vi "CI Project Builder.vi"() -> ()   [LabVIEW 2014, in "CI Project Builder.lvlib"]
doc: "This is the main VI for the configuration editor."
uses:
  CI Project Builder.lvlib
  Controls/StateCluster.ctl
  <vilib>/ni/Configuration Framework/Node/NodeRef.ctl
  <vilib>/ni/Configuration Framework/Node/NISE_CEF_Node.lvclass
  <vilib>/ni/Configuration Framework/Node/StandardEvents.ctl
  <vilib>/ni/Configuration Framework/Node/UserEventRef.ctl
  <vilib>/ni/Configuration Framework/Controls/EventCluster.ctl
  <vilib>/ni/Configuration Framework/Node/NodeChangeEvent.ctl
  <vilib>/ni/Configuration Framework/Node/CacheState.ctl
  <vilib>/ni/Configuration Framework/Node/RefreshUIEvent.ctl
  <vilib>/ni/Configuration Framework/Node/StopEvent.ctl
  <vilib>/ni/Configuration Framework/glyph manager/glyph manager.ctl
  <vilib>/picture/picture.llb/imagedata.ctl
  Controls/AddMessage.ctl
  Controls/MoveMessage.ctl
  <vilib>/Utility/error.llb/DialogType.ctl
  <vilib>/ni/AMC/Message Queue.ctl
  <vilib>/ni/AMC/Message.ctl
  <vilib>/ni/Tools/Keyed Array/KeyedArray.ctl
  Classes/CI Project/CI Project.lvclass
  <vilib>/ni/Configuration Framework/class discovery singleton/class discovery singleton methods.ctl
  <vilib>/ni/AMC/Read Termination Message.vi
  <vilib>/ni/AMC/Create Single Message.vi
  <vilib>/ni/AMC/Update Message Routing Info.vi
  <vilib>/ni/AMC/Send Message.vi
  <vilib>/ni/AMC/Globals.vi
  Classes/INI Deserializer/INI Deserializer.lvclass
  <vilib>/ni/AMC/AMC.lvlib
  <vilib>/ni/Configuration Framework/NISE_CEF_TreeControl.lvlib
  <vilib>/ni/Configuration Framework/glyph manager/glyph manager.lvlib
  <vilib>/ni/Configuration Framework/class discovery singleton/class discovery singleton.lvlib
  <vilib>/ni/Tools/Keyed Array/Tools_KeyedArray.lvlib
panel:
  in  "View":string(tree)
  in  "Exit":bool
  # "Continuous Integration Project Builder"
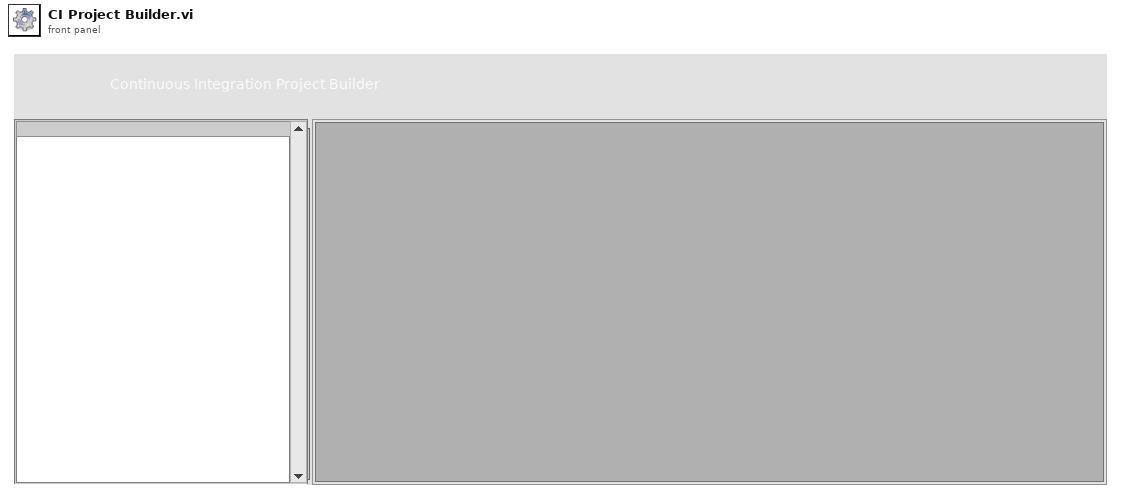
[diagram p1: front panel]
types:
  T1 = typedef "CI Project Builder.lvlib/StateCluster.ctl" = cluster{"root":T2, "unsaved changes":bool, "current path":path, "standard events":T3, "classes path":path, "glyph manager":T9, "Exports Path":path}
  T2 = typedef "NISE_CEF_Node.lvclass/NodeRef.ctl" = refnum<data-value>
  T3 = typedef "NISE_CEF_Node.lvclass/StandardEvents.ctl" = cluster{"user event":T4, "node change":T5, "cache state":T6, "refresh UI":T7, "stop event":T8}
  T4 = typedef "NISE_CEF_Node.lvclass/UserEventRef.ctl" = refnum<user-event>
  T5 = typedef "NISE_CEF_Node.lvclass/NodeChangeEvent.ctl" = refnum<user-event>
  T6 = typedef "NISE_CEF_Node.lvclass/CacheState.ctl" = refnum<user-event>
  T7 = typedef "NISE_CEF_Node.lvclass/RefreshUIEvent.ctl" = refnum<user-event>
  T8 = typedef "NISE_CEF_Node.lvclass/StopEvent.ctl" = refnum<user-event>
  T9 = typedef "glyph manager.lvlib/glyph manager.ctl" = cluster{"search paths":path[], "glyph map":variant, "base glyphs":T10[], "desired overlays":string[]}
  T10 = typedef "imagedata.ctl" = cluster{"image type":i32, "image depth":i32, "image":u8[], "mask":u8[], "colors":u32[], "Rectangle":cluster{"left":i16, "top":i16, "right":i16, "bottom":i16}}
  T11 = typedef "AMC.lvlib/Message Queue.ctl" = refnum<queue>
  T12 = enum32{"Invalid", "Standard", "Closed", "Hidden", "Minimized", "Maximized"}
  T13 = typedef "class discovery singleton.lvlib/class discovery singleton methods.ctl" = enum16{"add search paths", "load class by name", "list available classes", "get class path", "delete cache"}
  T14 = typedef "CI Project Builder.lvlib/AddMessage.ctl" = cluster{"node type":string, "to add to":string}
  T15 = typedef "CI Project Builder.lvlib/MoveMessage.ctl" = cluster{"node ref":T2, "new parent":T2, "Position":i32}
  T16 = typedef "CI Project Builder.lvlib/FilePaths.ctl" = cluster{"glyphs":path, "classes":path}
  T17 = typedef "DialogType.ctl" = u16
  T18 = typedef "NISE_CEF_Node.lvclass/Summary.ctl" = cluster{"ID":string, "parent ID":string, "node type":string, "text":string, "additional text":string, "glyph":string, "depth":i32, "glyph overlay":string}
  T19 = typedef "LVPoint32TypeDef.ctl" = cluster{"Horizontal":i32, "Vertical":i32}
  T20 = cluster{"data name":string, "drag data":variant}[]
  T21 = typedef "NISE_CEF_Node.lvclass/NodeMenuOptions.ctl" = cluster{"removable":bool, "movable":bool, "duplicate":bool}
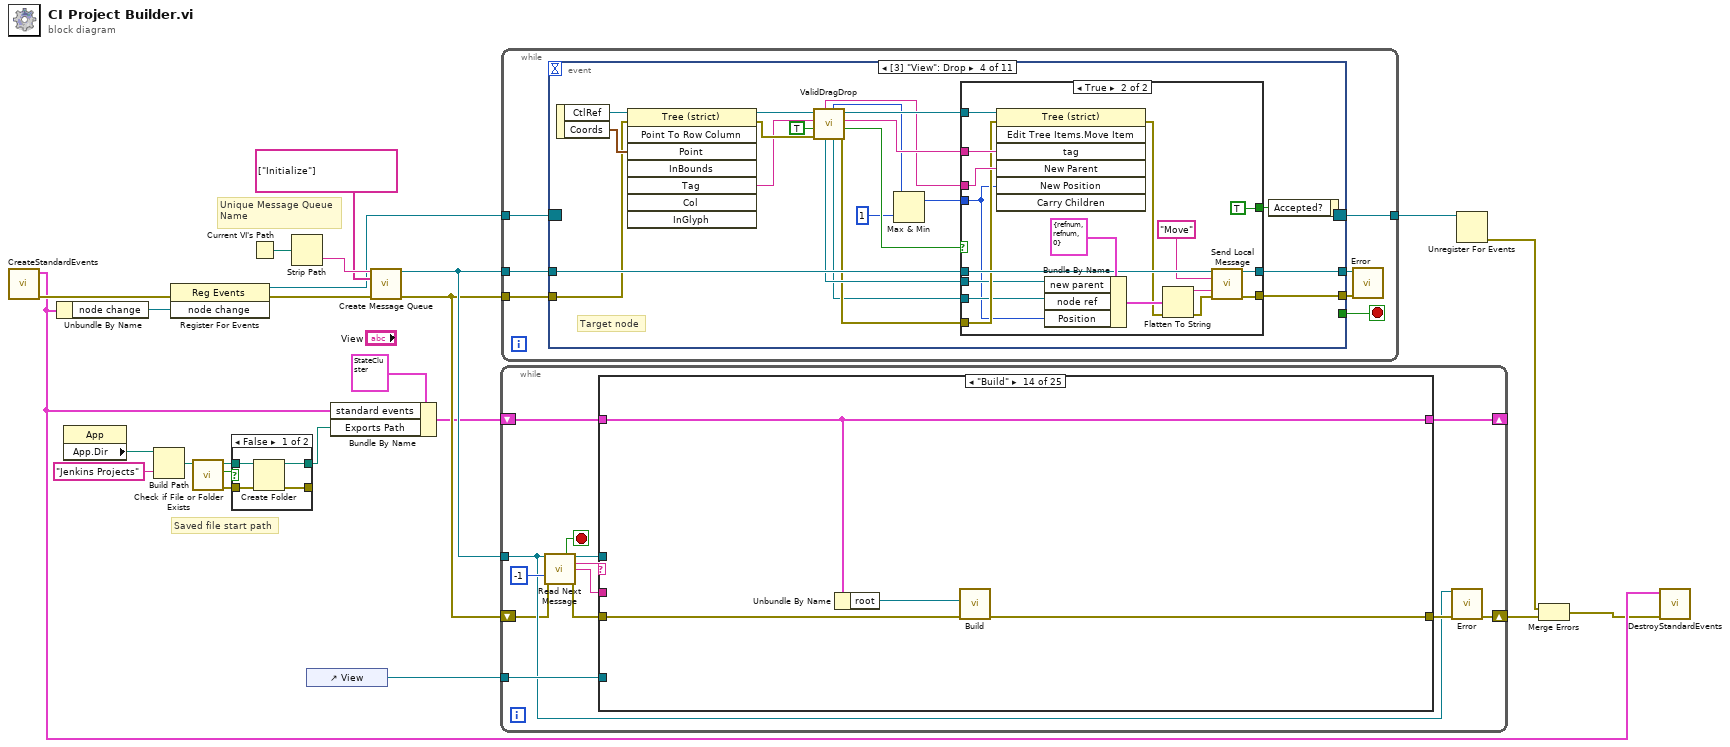
[diagram p0: block diagram]
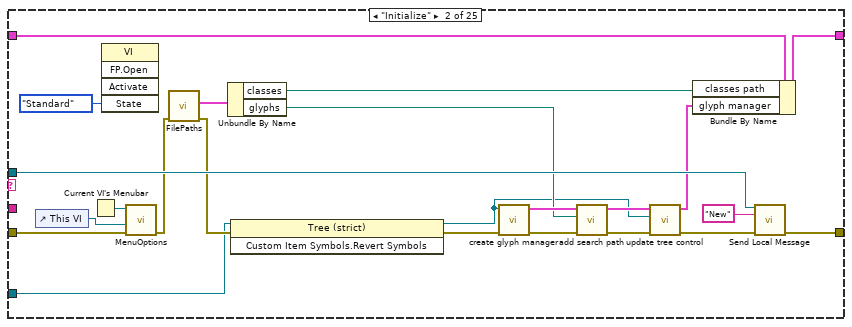
[diagram p4: hidden frame]
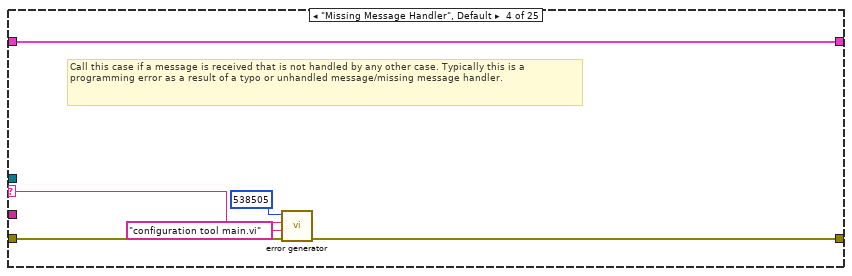
[diagram p6: hidden frame]
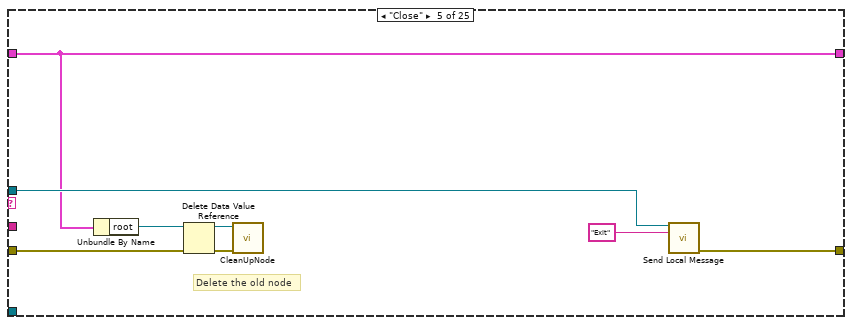
[diagram p7: hidden frame]
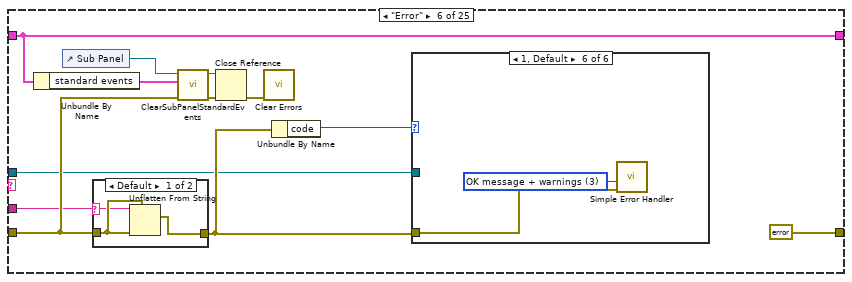
[diagram p8: hidden frame]
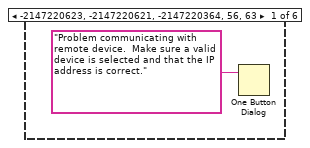
[diagram p10: hidden frame]
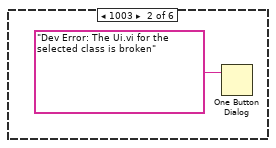
[diagram p11: hidden frame]
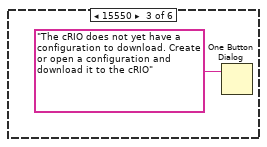
[diagram p12: hidden frame]
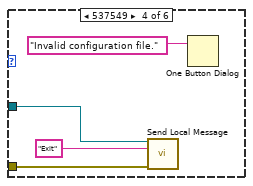
[diagram p13: hidden frame]
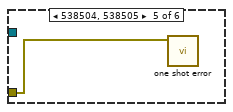
[diagram p14: hidden frame]
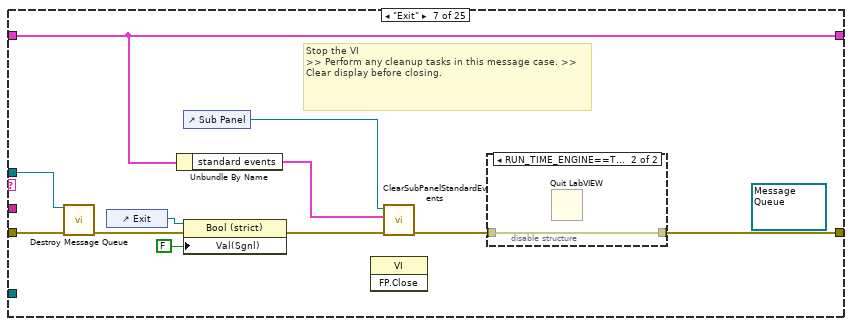
[diagram p15: hidden frame]
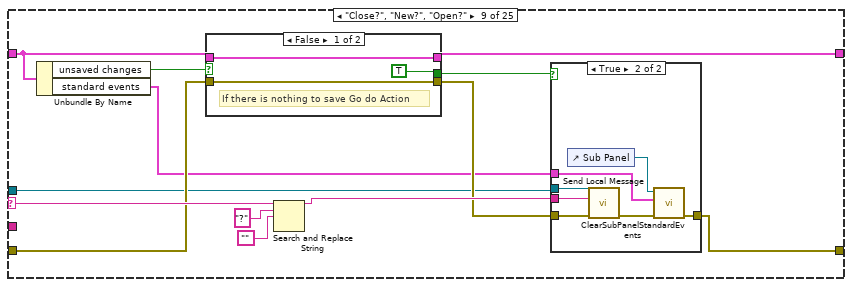
[diagram p18: hidden frame]
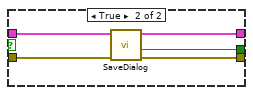
[diagram p19: hidden frame]
diagram:
  # "Saved file start path"
  # "Unique Message Queue Name"
  n1 = call <vilib>:"CreateStandardEvents.vi"() -> ("error out"=w19:errorcluster, "standard events"=w13:T3)  [unwired: 10 in]
  n2 = Unbundle By Name(w13) -> ("node change"=w18:T5)
  n3 = property class="App"() -> ("App.Dir"=w2:path)  [unwired: 2 in, 2 out]
  n4 = Build Path(base path=w2, name or relative path="Jenkins Projects") -> (appended path=w3:path)
  n5 = register-events(error in=w19, w18) -> (reference out=w12:refnum<event-registration>, error out=w17:errorcluster)  [unwired: 1 in]
  n6 = call <vilib>:"Check if File or Folder Exists.vi"("path"=w3) -> ("error out"=w4:errorcluster, "file or folder exists?"=w6:bool, "dup path"=w5:path)  [unwired: 8 in]
  n7 = case shown="False" w6 {
    tunnel: w5 -> [w28 w30]
    tunnel: [w27 w30] -> w1
    tunnel: w4 -> [w26 w29]
    tunnel: [w25 w29] -> _
    frame False {
      n8 = Create Folder(path (use dialog)=w28, error in=w26) -> (created path=w27:path, error out=w25:errorcluster)  [unwired: 1 in, 1 out]
    }
    frame True {
    }
  }
  n9 = Current VI's Path() -> (path=w23:path)
  n10 = Strip Path(path=w23) -> (name=w24:string)  [unwired: 1 out]
  n11 = control-ref of="View"() -> (w11:refnum<vi>)
  n12 = Bundle By Name(cluster=T1 {"root"=refnum, "unsaved changes"=FALSE, "current path"=path "", "standard events"={"user event"=refnum, "node change"=refnum, "cache state"=refnum, "refresh UI"=refnum, "stop event"=refnum}, "classes path"=path "", "glyph manager"={"search paths"=[], "glyph map"=variant, "base glyphs"=[], "desired overlays"=[]}, "Exports Path"=path ""}, "standard events"=w13, "Exports Path"=w1) -> (w15:T1)
  n13 = call <vilib>:"Create Message Queue.vi"("message queue name"=w24, "initial message names"=string[] ["Initialize"], "error in"=w17) -> ("message queue out"=w21:T11, "error out"=w20:errorcluster)  [unwired: 11 in]
  n14 = while "Message Processor" {
    shift-right: [w34] -> w14
    shift-left: w20 -> [w32]
    tunnel: w21 -> [w33]
    shift-right: [w40] -> _
    shift-left: w15 -> [w39]
    tunnel: w11 -> [w37]
    stop <- w43 stop-if-true
    n15 = call <vilib>:"Read Next Message.vi"("message queue in"=w33, "timeout (1 ms)"=-1, "error in"=w32) -> ("exit process?"=w43:bool, "message queue out"=w38:T11, "message name"=w42:string, "message value"=w41:string, "error out"=w31:errorcluster)  [unwired: 5 in, 3 out]
    n16 = case shown="\"Build\"" w42 {
      selector: w42 -> [_ _ _ w72 _ _ _ _ w135 _ _ _ _ _ _ _ _ w284 _ _ _ _ _ _ _]
      tunnel: w41 -> [_ _ _ _ _ w87 _ _ _ _ _ _ _ _ _ w251 w262 w282 w335 w361 _ _ w401 w424 w429]
      tunnel: w31 -> [w45 w68 w70 w75 w79 w90 w121 w125 w128 w157 w175 w204 w219 w224 w227 w232 w261 w287 w337 w360 w382 w391 w400 w422 w430]
      tunnel: [w45 w64 w70 w73 w83 errorcluster {"status"=FALSE, "code"=0, "source"=""} ("error out") w113 w125 w138 w169 w171 w206 w221 w223 w227 w245 w265 w290 w339 w357 w376 w387 w397 w417 w428] -> w35
      tunnel: [w44 w60 w69 w76 w81 w94 w112 w124 w130 w167 w176 w209 w220 w225 w226 w242 w258 w291 w338 w354 w373 w390 w396 w413 w431] -> w40
      tunnel: w39 -> [w44 w61 w69 w76 w81 w94 w112 w124 w131 w164 w177 w201 w218 w225 w226 w233 w259 w291 w331 w362 w385 w390 w396 w425 w431]
      tunnel: w38 -> [_ w63 _ _ w82 w85 w120 _ w126 w168 w173 w205 _ _ _ _ _ w285 _ _ _ _ w393 w416 w427]
      tunnel: w37 -> [_ w47 _ _ _ _ _ _ _ _ _ _ _ _ _ w243 w254 w279 w333 w355 w374 _ _ _ _]
      frame "------------Generic Operations------------" {
        # "Dummy case to add a seperation in the Case Structure menu"
      }
      frame "Initialize" {
        n17 = control-ref of="This VI"() -> (w67:refnum<vi>)
        n18 = Current VI's Menubar() -> (w66:refnum<k9>)
        n19 = invoke class="VI" method="FP.Open"("State"=T12."Standard") -> ()  [unwired: 4 in, 5 out]
        n20 = call "MenuOptions.vi"("error in"=w68, "VI ref"=w67, "menu ref in"=w66) -> ("error out"=w59:errorcluster)  [unwired: 7 in, 1 out]
        n21 = call "FilePaths.vi"("error in"=w59) -> ("error out"=w50:errorcluster, "paths"=w62:T16)  [unwired: 9 in]
        n22 = Unbundle By Name(w62) -> ("classes"=w58:path, "glyphs"=w52:path)
        n23 = invoke class="Tree (strict)" method="Custom Item Symbols.Revert Symbols"(reference=w47, error in=w50) -> (reference out=w48:refnum<vi>, error out=w49:errorcluster)  [unwired: 1 in, 1 out]
        n24 = call <vilib>:"create glyph manager.vi"("error in"=w49, "tree ref (for default symbols)"=w48) -> ("error out"=w57:errorcluster, "glyph manager"=w56:T9)  [unwired: 8 in]
        n25 = call <vilib>:"add search path.vi"("error in"=w57, "search path"=w52, "glyph manager in"=w56) -> ("error out"=w55:errorcluster, "glyph manager out"=w54:T9)  [unwired: 7 in]
        n26 = call <vilib>:"update tree control.vi"("error in"=w55, "tree reference"=w48, "glyph manager in"=w54) -> ("error out"=w53:errorcluster, "glyph manager out"=w51:T9)  [unwired: 7 in]
        n27 = Bundle By Name(cluster=w61, "classes path"=w58, "glyph manager"=w51) -> (w60:T1)
        n28 = call <vilib>:"Send Local Message.vi"("message queue in"=w63, "message name"="New" ("Message Name"), "error in"=w53) -> ("error out"=w64:errorcluster)  [unwired: 10 in, 2 out]
      }
      frame "", "Idle" {
      }
      frame "Missing Message Handler", Default {
        # "Call this case if a message is received that is not handled by any other case. Typically this is a programming error as a result of a typo or unhandled message/missing message handler."
        n29 = call <vilib>:"error generator.vi"("error in"=w75, "source"="configuration tool main.vi", "append error message"=w72, "error code (0)"=538505) -> ("error out"=w73:errorcluster)  [unwired: 5 in]
      }
      frame "Close" {
        # "Delete the old node"
        n30 = Unbundle By Name(w81) -> ("root"=w80:T2)
        n31 = Delete Data Value Reference(data value reference=w80, error in=w79) -> (data value=w78:refnum<class "NISE_CEF_Node.lvclass">, error out=w77:errorcluster)
        n32 = call-dynamic "CleanUpNode.vi"("error in (no error)"=w77, "NISE_CEF_Node in"=w78) -> ()  [unwired: 8 in, 2 out]
        n33 = call <vilib>:"Send Local Message.vi"("message queue in"=w82, "message name"="Exit") -> ("error out"=w83:errorcluster)  [unwired: 11 in, 2 out]
      }
      frame "Error" {
        n34 = Unbundle By Name(w94) -> ("standard events"=w86:T3)
        n35 = control-ref of="Sub Panel"() -> (w93:refnum<vi>)
        n36 = case shown="Default" w87 {
          selector: w87 -> [w98 _]
          tunnel: w90 -> [w99 w100]
          tunnel: [w97 w100] -> w89
          frame Default {
            n37 = Unflatten From String(type=w99, binary string=w98, error in (no error)=w99) -> (value=w97:errorcluster)  [unwired: 2 in, 2 out]
          }
          frame "" {
          }
        }
        n38 = call <vilib>:"ClearSubPanelStandardEvents.vi"("error in"=w90, "standard events"=w86, "sub panel ref in"=w93) -> ("error out"=w92:errorcluster, "sub panel ref out"=w91:refnum<vi>)  [unwired: 7 in]
        n39 = Close Reference(reference=w91, error in (no error)=w92) -> (error out=w88:errorcluster)
        n40 = call <vilib>:"Clear Errors.vi"("error in (no error)"=w88) -> ()  [unwired: 5 in, 2 out]
        n41 = Unbundle By Name(w89) -> ("code"=w95:i32)
        n42 = case shown="1, Default" w95 {
          tunnel: w85 -> [_ _ _ w106 _ _]
          tunnel: w89 -> [_ _ _ w105 w108 w110]
          frame -2147220623, -2147220621, -2147220364, 56, 63 {
            n43 = One Button Dialog(message="Problem communicating with remote device.  Make sure a valid device is selected and that the IP address is correct.") -> ()  [unwired: 1 in, 1 out]
          }
          frame 1003 {
            n44 = One Button Dialog(message="Dev Error: The Ui.vi for the selected class is broken") -> ()  [unwired: 1 in, 1 out]
          }
          frame 15550 {
            n45 = One Button Dialog(message="The cRIO does not yet have a configuration to download. Create or open a configuration and download it to the cRIO") -> ()  [unwired: 1 in, 1 out]
          }
          frame 537549 {
            n46 = call <vilib>:"Send Local Message.vi"("message queue in"=w106, "message name"="Exit", "error in"=w105) -> ()  [unwired: 10 in, 3 out]
            n47 = One Button Dialog(message="Invalid configuration file.") -> ()  [unwired: 1 in, 1 out]
          }
          frame 538504, 538505 {
            n48 = call <vilib>:"one shot error.vi"("error in"=w108) -> ()  [unwired: 11 in]
          }
          frame 1, Default {
            w109 = T17 3 items=["no dialog", "OK message", "continue or stop message", "OK message + warnings", "continue/stop + warnings"] ("type of dialog (OK msg:1)")
            n49 = call <vilib>:"Simple Error Handler.vi"("type of dialog (OK msg:1)"=w109, "error in (no error)"=w110) -> ()  [unwired: 8 out]
          }
        }
      }
      frame "Exit" {
        (unwired) T11 refnum ("message queue out")
        # "Stop the VI                                                                             >> Perform any cleanup tasks in this message case. >> Clear display before closing."
        n50 = call <vilib>:"Destroy Message Queue.vi"("message queue in"=w120, "error in"=w121) -> ("error out"=w117:errorcluster)  [unwired: 11 in, 2 out]
        n51 = control-ref of="Exit"() -> (w119:refnum<vi>)
        n52 = Unbundle By Name(w112) -> ("standard events"=w111:T3)
        n53 = control-ref of="Sub Panel"() -> (w116:refnum<vi>)
        n54 = property class="Bool (strict)"(reference=w119, error in=w117, "Val(Sgnl)"=FALSE ("Exit")) -> (error out=w115:errorcluster)  [unwired: 1 out]
        n55 = invoke class="VI" method="FP.Close"() -> ()  [unwired: 3 in, 3 out]
        n56 = call <vilib>:"ClearSubPanelStandardEvents.vi"("error in"=w115, "standard events"=w111, "sub panel ref in"=w116) -> ("error out"=w114:errorcluster)  [unwired: 7 in, 1 out]
        n57 = disable-structure shown="RUN_TIME_ENGINE==True" {
          disable-tunnel: [w122 w123] -> w113
          disable-tunnel: w114 -> [w122 w123]
          frame condition #0 (active) {
          }
          frame condition #1 {
            n58 = Quit LabVIEW() -> ()  [unwired: 1 in]
          }
        }
      }
      frame "------------Menu Operations--------------" {
        # "Dummy case to add a seperation in the Case Structure menu"
      }
      frame "Close?", "New?", "Open?" {
        n59 = Unbundle By Name(w131) -> ("unsaved changes"=w133:bool, "standard events"=w127:T3)
        n60 = case shown="False" w133 {
          tunnel: [TRUE ("SaveFlag") w146] -> w132
          tunnel: w131 -> [w140 w145]
          tunnel: [w140 w144] -> w130
          tunnel: w128 -> [w139 w143]
          tunnel: [w139 w142] -> w129
          frame False {
            # "If there is nothing to save Go do Action"
          }
          frame True {
            n61 = call "SaveDialog.vi"("error in"=w143, "state in"=w145) -> ("error out"=w142:errorcluster, "new"=w146:bool, "state out"=w144:T1)  [unwired: 7 in]
          }
        }
        n62 = Search and Replace String(input string=w135, search string="?", replace string="") -> (result string=w134:string)  [unwired: 5 in, 3 out]
        n63 = case shown="True" w132 {
          tunnel: w129 -> [w147 w154]
          tunnel: [w147 w150] -> w138
          tunnel: w126 -> [_ w153]
          tunnel: w134 -> [_ w152]
          tunnel: w127 -> [_ w148]
          frame False {
          }
          frame True {
            n64 = control-ref of="Sub Panel"() -> (w149:refnum<vi>)
            n65 = call <vilib>:"Send Local Message.vi"("message queue in"=w153, "message name"=w152, "error in"=w154) -> ("error out"=w151:errorcluster)  [unwired: 10 in, 2 out]
            n66 = call <vilib>:"ClearSubPanelStandardEvents.vi"("error in"=w151, "standard events"=w148, "sub panel ref in"=w149) -> ("error out"=w150:errorcluster)  [unwired: 7 in, 1 out]
          }
        }
      }
      frame "New" {
        # "Delete the old node, if any"
        n67 = Unbundle By Name(w164) -> ("root"=w156:T2, "classes path"=w159:path)
        n68 = Delete Data Value Reference(data value reference=w156) -> (data value=w155:refnum<class "NISE_CEF_Node.lvclass">)  [unwired: 1 in, 1 out]
        n69 = call-dynamic "CleanUpNode.vi"("NISE_CEF_Node in"=w155) -> ()  [unwired: 9 in, 2 out]
        n70 = Build Array(w159) -> (w160:path[])
        n71 = call <vilib>:"class discovery singleton.vi"("error in"=w157, "Plugin Search Paths"=w160, "method"=class_discovery_singleton_methods."add search paths") -> ("error out"=w158:errorcluster)  [unwired: 5 in, 3 out]
        n72 = call-dynamic "Initialize.vi"("error in"=w158, "node in"=refnum<class "CI Project.lvclass"> refnum ("CI Project.lvclass")) -> ("error out"=w163:errorcluster, "data value reference"=w165:T2)  [unwired: 7 in, 1 out]
        n73 = Bundle By Name(cluster=w164, "unsaved changes"=FALSE ("SaveFlag"), "root"=w165) -> (w167:T1)
        n74 = call <vilib>:"Send Local Message.vi"("message queue in"=w168, "message name"="PopulateTree", "error in"=w163) -> ("error out"=w169:errorcluster)  [unwired: 10 in, 2 out]
      }
      frame "Open" {
        # "Delete the old node"
        n75 = in-place {
          in-place-border: w175 -> [w186]
          in-place-border: [w185] -> w172
          n76 = in-place-cluster #1(w177) -> ("current path"=w183:path, "root"=w187:T2, "Exports Path"=w178:path)  [unwired: 1 out]
          n77 = call "FileDialog.vi"("error in"=w186, "start path"=w178) -> ("error out"=w180:errorcluster, "cancelled"=w181:bool, "selected path"=w184:path)  [unwired: 7 in]
          n78 = case shown="False" w181 {
            tunnel: [w191 w199] -> w185
            tunnel: [w195 w200] -> w179
            tunnel: w184 -> [w198 _]
            tunnel: w180 -> [w197 w199]
            tunnel: w187 -> [w189 w200]
            frame False {
              n79 = Delete Data Value Reference(data value reference=w189) -> (data value=w190:refnum<class "NISE_CEF_Node.lvclass">)  [unwired: 1 in, 1 out]
              n80 = call-dynamic "CleanUpNode.vi"("NISE_CEF_Node in"=w190) -> ()  [unwired: 9 in, 2 out]
              n81 = call "Open.vi"("error in (no error)"=w197, "INI Path"=w198) -> ("error out"=w196:errorcluster, "INI Deserializer out"=w193:refnum<class "INI Deserializer.lvclass">)  [unwired: 8 in]
              n82 = call-dynamic "Deserialize.vi"("error in (no error)"=w196, "CI Deserializer in"=w193) -> ("error out"=w194:errorcluster, "CI Deserializer out"=w192:refnum<class "INI Deserializer.lvclass">, "Node out"=w195:T2)  [unwired: 7 in]
              n83 = call "Close.vi"("error in (no error)"=w194, "INI Deserializer in"=w192) -> ("error out"=w191:errorcluster)  [unwired: 9 in]
            }
            frame True {
            }
          }
          n84 = Select(t=w183, s=w185, f=w184) -> (s? t:f=w182:path)
          n85 = in-place-cluster #1("current path"=w182, "unsaved changes"=FALSE ("SaveFlag"), "root"=w179, "Exports Path"=w178) -> (w176:T1)
        }
        n86 = call <vilib>:"Send Local Message.vi"("message queue in"=w173, "message name"="PopulateTree", "error in"=w172) -> ("error out"=w171:errorcluster)  [unwired: 10 in, 2 out]
      }
      frame "Save" {
        n87 = Unbundle By Name(w201) -> ("current path"=w203:path)
        n88 = Empty String/Path?(string/path=w203) -> (empty?=w202:bool)
        n89 = case shown="False" w202 {
          tunnel: w201 -> [w213 w215]
          tunnel: [w212 w214] -> w209
          tunnel: [w211 w216] -> w207
          tunnel: w204 -> [w210 w217]
          frame False {
            n90 = call "Save.vi"("error in"=w210, "state in"=w213) -> ("error out"=w211:errorcluster, "state out"=w212:T1)  [unwired: 8 in]
          }
          frame True {
            # "Empty path use Dialog"
            n91 = call "SaveAs.vi"("error in"=w217, "state in"=w215) -> ("error out"=w216:errorcluster, "state out"=w214:T1)  [unwired: 7 in, 1 out]
          }
        }
        n92 = call <vilib>:"Send Local Message.vi"("message queue in"=w205, "message name"="PopulateTree", "error in"=w207) -> ("error out"=w206:errorcluster)  [unwired: 10 in, 2 out]
      }
      frame "SaveAs" {
        n93 = call "SaveAs.vi"("error in"=w219, "state in"=w218) -> ("error out"=w221:errorcluster, "state out"=w220:T1)  [unwired: 7 in, 1 out]
      }
      frame "Build" {
        n94 = Unbundle By Name(w225) -> ("root"=w222:T2)
        n95 = call "Build.vi"("error in (no error)"=w224, "Root Node"=w222) -> ("error out"=w223:errorcluster)  [unwired: 9 in]
      }
      frame "-------TreeControl Operations-----------" {
        # "Dummy case to add a seperation in the Case Structure menu"
      }
      frame "AddNode" {
        n96 = Unflatten From String(type=T14 {"node type"="", "to add to"=""} ("input cluster"), binary string=w251) -> (value=w249:T14)  [unwired: 3 in, 2 out]
        n97 = Unbundle By Name(w249) -> ("to add to"=w247:string, "node type"=w230:string)
        n98 = call <vilib>:"class discovery singleton.vi"("error in"=w232, "Class Name"=w230, "method"=class_discovery_singleton_methods."get class path") -> ("error out"=w231:errorcluster, "class path"=w229:path)  [unwired: 5 in, 2 out]
        n99 = Unbundle By Name(w233) -> ("glyph manager"=w239:T9)
        n100 = call <vilib>:"Get LV Class Default Value.vi"("error in (no error)"=w231, "class path"=w229) -> ("error out"=w252:errorcluster, "object"=w253:refnum<class>)  [unwired: 8 in]
        n101 = To More Specific Class(target class=refnum<class "NISE_CEF_Node.lvclass"> refnum ("Node.lvclass"), reference=w253, error in=w252) -> (specific class reference=w240:refnum<class "NISE_CEF_Node.lvclass">, error out=w241:errorcluster)
        n102 = call-dynamic "AddGlyphtoGManager.vi"("error in"=w241, "glyph manager"=w239, "NISE_CEF_Node in"=w240) -> ("error out"=w237:errorcluster, "glyph manager out"=w238:T9, "NISE_CEF_Node out"=w236:refnum<class "NISE_CEF_Node.lvclass">)  [unwired: 6 in]
        n103 = call <vilib>:"AddNode.vi"("error in"=w237, "node in"=w236, "parent node ID"=w247) -> ("error out"=w246:errorcluster, "summary"=w244:T18[])  [unwired: 7 in]
        n104 = call <vilib>:"PopulateTreeSumaryWithGlyphManager.vi"("error in"=w246, "glyph manager"=w238, "summary"=w244, "tree ref in"=w243) -> ("error out"=w245:errorcluster, "glyph manager out"=w235:T9)  [unwired: 6 in]
        n105 = Bundle By Name(cluster=w233, "glyph manager"=w235, "unsaved changes"=TRUE) -> (w242:T1)
      }
      frame "Duplicate" {
        n106 = call <vilib>:"IDtoNode.vi"("error in"=w261, "ID"=w262) -> ("error out"=w263:errorcluster, "invalid Id"=w260:bool, "node ref"=w264:T2)  [unwired: 7 in]
        n107 = Unbundle By Name(w259) -> ("glyph manager"=w256:T9)
        n108 = case shown="False" w260 {
          tunnel: [w276 w278] -> w265
          tunnel: w264 -> [w275 _]
          tunnel: w263 -> [w272 w278]
          tunnel: w256 -> [w268 w277]
          tunnel: [w267 w277] -> w255
          tunnel: w254 -> [w266 _]
          frame False {
            n109 = call <vilib>:"DuplicateNode.vi"("same parent?"=TRUE ("s"), "error in"=w272, "node ref in"=w275) -> ("error out"=w273:errorcluster, "new node ref"=w274:T2)  [unwired: 7 in]
            n110 = call <vilib>:"Summary.vi"("error in"=w273, "node self ref"=w274) -> ("error out"=w270:errorcluster, "summary"=w269:T18[])  [unwired: 8 in]
            n111 = call <vilib>:"PopulateTreeSumaryWithGlyphManager.vi"("error in"=w270, "glyph manager"=w268, "summary"=w269, "tree ref in"=w266) -> ("error out"=w276:errorcluster, "glyph manager out"=w267:T9)  [unwired: 6 in]
          }
          frame True {
          }
        }
        n112 = Bundle By Name(cluster=w259, "unsaved changes"=TRUE, "glyph manager"=w255) -> (w258:T1)
      }
      frame "CustomMenuAction" {
        n113 = Match Pattern(string=w282, regular expression=":") -> (before substring=w281:string, after substring=w280:string)  [unwired: 1 in, 2 out]
        n114 = call <vilib>:"IDtoNode.vi"("error in"=w287, "ID"=w280) -> ("error out"=w288:errorcluster, "invalid Id"=w286:bool, "node ref"=w289:T2)  [unwired: 7 in]
        n115 = case shown="False" w286 {
          tunnel: [w298 w327] -> w290
          tunnel: w289 -> [w295 _]
          tunnel: w288 -> [w301 w327]
          tunnel: w285 -> [w292 _]
          tunnel: w284 -> [_ _]
          tunnel: w281 -> [w299 _]
          tunnel: w279 -> [w296 _]
          frame False {
            n116 = in-place {
              in-place-border: w292 -> [w325]
              in-place-border: w301 -> [w323]
              in-place-border: [w322] -> w297
              in-place-border: [w321] -> w300
              in-place-border: w299 -> [w320]
              in-place-border: w296 -> [w319]
              in-place-border: [w318] -> w294
              n117 = in-place-dvr #2(w295) -> (w326:refnum<class "NISE_CEF_Node.lvclass">)  [unwired: 1 out]
              n118 = call-dynamic "MenuHandler.vi"("tree control"=w319, "main message queue"=w325, "error in"=w323, "menu string"=w320, "NISE_CEF_Node in"=w326) -> ("error out"=w322:errorcluster, "refresh tree?"=w318:bool, "Unhandled"=w321:bool, "NISE_CEF_Node out"=w324:refnum<class "NISE_CEF_Node.lvclass">)  [unwired: 3 in]
              n119 = in-place-dvr #2(w324) -> (w293:T2)  [unwired: 1 out]
            }
            n120 = case shown="False" w300 {
              tunnel: w299 -> [_ w313]
              tunnel: [w305 w314] -> w298
              tunnel: w297 -> [w303 w315]
              tunnel: w294 -> [w302 _]
              tunnel: w293 -> [w304 _]
              frame False {
                n121 = case shown="False" w302 {
                  tunnel: [w306 w309] -> w305
                  tunnel: w304 -> [_ w308]
                  tunnel: w303 -> [w306 w307]
                  frame False {
                  }
                  frame True {
                    n122 = call <vilib>:"NodetoID.vi"("error in"=w307, "node ref"=w308) -> ("error out"=w311:errorcluster, "ID"=w312:string)  [unwired: 8 in]
                    n123 = call <vilib>:"Send Local Message.vi"("message name"="NodeDataChange", "message value"=w312, "error in"=w311) -> ("error out"=w309:errorcluster)  [unwired: 10 in, 2 out]
                  }
                }
              }
              frame True {
                n124 = call <vilib>:"error generator.vi"("error in"=w315, "source"="configuration tool main.vi", "append error message"=w313, "error code (0)"=538506) -> ("error out"=w314:errorcluster)  [unwired: 5 in]
              }
            }
          }
          frame True {
          }
        }
      }
      frame "RefreshNode" {
        # "Refreshes the node in the Tree, Sets the save flag to true. This case can be called from the UIs of the nodes"
        n125 = Unbundle By Name(w331) -> ("glyph manager"=w330:T9)
        n126 = call <vilib>:"IDtoNode.vi"("error in"=w337, "ID"=w335) -> ("error out"=w336:errorcluster, "invalid Id"=w329:bool, "node ref"=w334:T2)  [unwired: 7 in]
        n127 = case shown="False" w329 {
          tunnel: [w349 w352] -> w339
          tunnel: w336 -> [w345 w352]
          tunnel: w334 -> [w344 _]
          tunnel: w333 -> [w343 _]
          tunnel: [w342 w351] -> w332
          tunnel: w330 -> [w340 w351]
          frame False {
            n128 = call <vilib>:"SummaryWithGlyphManager.vi"("error in"=w345, "glyph manager"=w340, "node self ref"=w344) -> ("error out"=w347:errorcluster, "glyph manager out"=w341:T9, "summary"=w346:T18[])  [unwired: 6 in]
            n129 = call <vilib>:"RefreshSubTreeWithGlyphManager.vi"("error in"=w347, "glyph manager"=w341, "node information"=w346, "tree ref in"=w343) -> ("error out"=w350:errorcluster, "glyph manager out"=w342:T9, "tree ref out"=w348:refnum<vi>)  [unwired: 5 in]
            n130 = Close Reference(reference=w348, error in (no error)=w350) -> (error out=w349:errorcluster)
          }
          frame True {
          }
        }
        n131 = Not(x=w329) -> (.not. x?=w328:bool)
        n132 = Bundle By Name(cluster=w331, "glyph manager"=w332, "unsaved changes"=w328) -> (w338:T1)
      }
      frame "RemoveNode" {
        n133 = call <vilib>:"IDtoNode.vi"("error in"=w360, "ID"=w361) -> ("error out"=w359:errorcluster, "invalid Id"=w356:bool, "node ref"=w358:T2)  [unwired: 7 in]
        n134 = case shown="False" w356 {
          tunnel: w359 -> [w368 w369]
          tunnel: w358 -> [w367 _]
          tunnel: [w364 w369] -> w357
          tunnel: w355 -> [w363 _]
          frame False {
            n135 = call <vilib>:"RemoveNode.vi"("error in"=w368, "node"=w367) -> ("error out"=w365:errorcluster, "node ID"=w366:string)  [unwired: 8 in]
            n136 = call <vilib>:"ClearTreeNode.vi"("error in"=w365, "tag"=w366, "tree reference"=w363) -> ("error out"=w364:errorcluster)  [unwired: 8 in]
          }
          frame True {
          }
        }
        n137 = Bundle By Name(cluster=w362, "unsaved changes"=TRUE) -> (w354:T1)
      }
      frame "PopulateTree" {
        n138 = Unbundle By Name(w385) -> ("standard events"=w375:T3, "glyph manager"=w371:T9, "root"=w380:T2)
        n139 = call <vilib>:"SummaryWithGlyphManager.vi"("error in"=w382, "glyph manager"=w371, "depth"=0 ("Depth"), "node self ref"=w380) -> ("error out"=w381:errorcluster, "glyph manager out"=w370:T9, "summary"=w384:T18[])  [unwired: 5 in]
        n140 = control-ref of="This VI"() -> (w383:refnum<vi>)
        n141 = call <vilib>:"RefreshEntireTreeWithGlyphManager.vi"("calling VI in"=w383, "error in"=w381, "glyph manager"=w370, "array"=w384, "tree ref in"=w374) -> ("error out"=w377:errorcluster, "glyph manager out"=w372:T9)  [unwired: 5 in]
        n142 = control-ref of="Sub Panel"() -> (w378:refnum<vi>)
        n143 = Bundle By Name(cluster=w385, "glyph manager"=w372) -> (w373:T1)
        n144 = call <vilib>:"ClearSubPanelStandardEvents.vi"("error in"=w377, "standard events"=w375, "sub panel ref in"=w378) -> ("error out"=w376:errorcluster)  [unwired: 7 in, 1 out]
      }
      frame "CleansubPanel" {
        # "Who else calls this case?"
        n145 = Unbundle By Name(w390) -> ("standard events"=w386:T3)
        n146 = control-ref of="Sub Panel"() -> (w392:refnum<vi>)
        n147 = call <vilib>:"ClearSubPanelStandardEvents.vi"("error in"=w391, "standard events"=w386, "sub panel ref in"=w392) -> ("error out"=w389:errorcluster, "sub panel ref out"=w388:refnum<vi>)  [unwired: 7 in]
        n148 = Close Reference(reference=w388, error in (no error)=w389) -> (error out=w387:errorcluster)
      }
      frame "ActivateNode" {
        n149 = Unbundle By Name(w396) -> ("standard events"=w395:T3)
        n150 = call <vilib>:"IDtoNode.vi"("error in"=w400, "ID"=w401) -> ("error out"=w394:errorcluster, "invalid Id"=w399:bool, "node ref"=w398:T2)  [unwired: 7 in]
        n151 = case shown="False" w399 {
          tunnel: w398 -> [w408 _]
          tunnel: [w409 w410] -> w397
          tunnel: w394 -> [w406 w410]
          tunnel: w393 -> [w404 _]
          tunnel: w395 -> [w402 _]
          frame False {
            n152 = control-ref of="Sub Panel"() -> (w405:refnum<vi>)
            n153 = call <vilib>:"ClearSubPanelStandardEvents.vi"("error in"=w406, "standard events"=w402, "sub panel ref in"=w405) -> ("error out"=w407:errorcluster, "sub panel ref out"=w403:refnum<vi>)  [unwired: 7 in]
            n154 = call <vilib>:"LoadNodeUIStandardEvents.vi"("user event out"=w402, "error in"=w407, "sub panel ref in"=w403, "main queue"=w404, "node"=w408) -> ("error out"=w409:errorcluster)  [unwired: 6 in]
          }
          frame True {
          }
        }
      }
      frame "Move" {
        n155 = Unflatten From String(type=T15 {"node ref"=refnum, "new parent"=refnum, "Position"=0} ("Cluster"), binary string=w424, error in (no error)=w422) -> (value=w421:T15, error out=w420:errorcluster)  [unwired: 2 in, 1 out]
        n156 = Unbundle By Name(w421) -> ("node ref"=w415:T2, "new parent"=w414:T2, "Position"=w411:i32)
        n157 = call <vilib>:"MoveNode.vi"("error in"=w420, "index"=w411, "new parent"=w414, "node"=w415) -> ("error out"=w418:errorcluster)  [unwired: 7 in]
        n158 = Bundle By Name(cluster=w425, "unsaved changes"=TRUE) -> (w413:T1)
        n159 = call <vilib>:"Send Local Message.vi"("message queue in"=w416, "message name"="PopulateTree", "error in"=w418) -> ("error out"=w417:errorcluster)  [unwired: 10 in, 2 out]
      }
      frame "NodeDataChange" {
        n160 = call <vilib>:"Send Local Message.vi"("message queue in"=w427, "message name"="RefreshNode", "message value"=w429, "error in"=w430) -> ("error out"=w428:errorcluster)  [unwired: 9 in, 2 out]
      }
    }
    n161 = call "Error.vi"("error in (no error)"=w35, "message queue in"=w33) -> ("error out"=w34:errorcluster)  [unwired: 9 in]
  }
  n162 = while "User Interface Event Handler" {
    tunnel: w21 -> [w438]
    tunnel: w20 -> [w434]
    tunnel: w12 -> [w433]
    tunnel: [w432] -> w8
    stop <- w437 stop-if-true
    n163 = event shown="[3] \"View\": Drop" {
      selector: w433 -> [_ _ _ _ _ _ _ _ _ _ _]
      dyn-events: [_ _ _ _ _ _ _ _ _ _ _] -> w432
      timeout: _ -> [_ _ _ _ _ _ _ _ _ _ _]
      tunnel: w438 -> [w440 w448 w472 w524 w553 w560 w589 w596 w604 w610 w652]
      tunnel: [_ _ _ _ TRUE _ _ _ _ _ _] -> w437
      tunnel: [w440 w448 w469 w522 w549 w560 w586 w596 w602 w609 w653] -> w436
      tunnel: [w439 w444 w468 w521 w550 w556 w585 w593 w600 w607 _] -> w435
      tunnel: w434 -> [w439 w447 w467 w523 w551 w559 w584 w595 w601 w608 _]
      event Timeout {
        # "Timeout code can be added here for autosave or Lock Screen"
        n164 = event-data() -> ()  [unwired: 1 in, 1 out]
      }
      event "View": Shortcut Menu Activation? {
        n165 = event-data() -> ("CtlRef"=w454:refnum<vi>, "Coords"=w453:T19, "MenuRef"=w450:refnum<k9>)  [unwired: 1 in]
        n166 = invoke class="Tree (strict)" method="Point To Row Column"(reference=w454, error in=w447, "Point"=w453) -> (error out=w446:errorcluster, "Tag"=w452:string)  [unwired: 5 in, 6 out]
        n167 = call <vilib>:"IDtoNode.vi"("error in"=w446, "ID"=w452) -> ("error out"=w442:errorcluster, "invalid Id"=w449:bool, "node ref"=w451:T2)  [unwired: 7 in]
        n168 = case shown="False" w449 {
          tunnel: w451 -> [w459 _]
          tunnel: w450 -> [w458 _]
          tunnel: [w457 _] -> w445
          tunnel: [w456 _] -> w443
          tunnel: w442 -> [w455 w465]
          tunnel: [w455 w465] -> w441
          frame False {
            n169 = in-place {
              in-place-border: w458 -> [w462]
              in-place-border: [w460] -> w457
              n170 = in-place-dvr #3(w459) -> (w464:refnum<class "NISE_CEF_Node.lvclass">, w461:errorcluster)
              n171 = call-dynamic "ShortcutMenu.vi"("error in"=w461, "menu ref in"=w462, "node in"=w464) -> ("error out"=w460:errorcluster, "node out"=w463:refnum<class "NISE_CEF_Node.lvclass">)  [unwired: 6 in, 1 out]
              n172 = in-place-dvr #3(w463) -> (w456:errorcluster)  [unwired: 1 out]
            }
          }
          frame True {
          }
        }
        n173 = Merge Errors(w443, w445, w441) -> (w444:errorcluster)
        n174 = event-data() -> ()  [unwired: 2 in, 1 out]
      }
      event "View": Shortcut Menu Selection (User) {
        n175 = event-data() -> ("ItemPath"=w471:string, "CtlRef"=w475:refnum<vi>, "Coords"=w476:T19)  [unwired: 1 in]
        n176 = invoke class="Tree (strict)" method="Point To Row Column"(reference=w475, error in=w467, "Point"=w476) -> (error out=w466:errorcluster, "Tag"=w470:string)  [unwired: 5 in, 6 out]
        n177 = Match Pattern(string=w471, regular expression=":") -> (before substring=w474:string, after substring=w473:string)  [unwired: 1 in, 2 out]
        n178 = case shown="\"Add\"" w474 {
          selector: w474 -> [w478 _ _ _]
          tunnel: w473 -> [_ _ _ w503]
          tunnel: w472 -> [w485 w492 w498 w505]
          tunnel: w470 -> [w480 w490 w496 w504]
          tunnel: [w482 w489 w495 w501] -> w469
          tunnel: [w483 w488 w493 w499] -> w468
          tunnel: w466 -> [w484 w487 w494 w500]
          frame Default {
            n179 = Concatenate Strings(w478, ":" ("string"), w480) -> (w481:string)
            n180 = call <vilib>:"Send Local Message.vi"("message queue in"=w485, "message name"="CustomMenuAction" ("Message Name"), "message value"=w481, "error in"=w484) -> ("message queue out"=w482:T11, "error out"=w483:errorcluster)  [unwired: 9 in, 1 out]
          }
          frame "Remove" {
            n181 = call <vilib>:"Send Local Message.vi"("message queue in"=w492, "message name"="RemoveNode" ("Message Name"), "message value"=w490, "error in"=w487) -> ("message queue out"=w489:T11, "error out"=w488:errorcluster)  [unwired: 9 in, 1 out]
          }
          frame "Duplicate" {
            n182 = call <vilib>:"Send Local Message.vi"("message queue in"=w498, "message name"="Duplicate" ("Message Name"), "message value"=w496, "error in"=w494) -> ("message queue out"=w495:T11, "error out"=w493:errorcluster)  [unwired: 9 in, 1 out]
          }
          frame "Add" {
            n183 = Bundle By Name(cluster=T14 {"node type"="", "to add to"=""} ("input cluster"), "node type"=w503, "to add to"=w504) -> (w506:T14)
            n184 = Flatten To String(anything=w506) -> (data string=w507:string)  [unwired: 3 in, 2 out]
            n185 = call <vilib>:"Send Local Message.vi"("message queue in"=w505, "message name"="AddNode" ("Message Name"), "message value"=w507, "error in"=w500) -> ("message queue out"=w501:T11, "error out"=w499:errorcluster)  [unwired: 9 in, 1 out]
          }
        }
      }
      event "View": Drop {
        # "Target node"
        n186 = event-data() -> ("CtlRef"=w527:refnum<vi>, "Coords"=w526:T19)  [unwired: 1 in]
        n187 = invoke class="Tree (strict)" method="Point To Row Column"(reference=w527, error in=w523, "Point"=w526) -> (reference out=w525:refnum<vi>, error out=w520:errorcluster, "Tag"=w516:string)  [unwired: 5 in, 5 out]
        n188 = call <vilib>:"ValidDragDrop.vi"("error in"=w520, "Reorder"=TRUE, "drag over"=w516, "Tree Ref in"=w525) -> ("Error Out"=w513:errorcluster, "Accepted"=w517:bool, "Drag"=w519:string, "Tree Ref out"=w529:refnum<vi>, "Moved Node"=w512:T2, "Position"=w511:i32, "Parent Node"=w518:T2, "Parent"=w515:string)
        n189 = Max & Min(x=w511, y=1) -> (max(x,y)=w514:i32)  [unwired: 1 out]
        n190 = case shown="True" w517 {
          tunnel: w519 -> [_ w546]
          tunnel: w529 -> [_ w548]
          tunnel: [_ TRUE] -> w528
          tunnel: w515 -> [_ w544]
          tunnel: w524 -> [w531 w543]
          tunnel: [w531 w540] -> w522
          tunnel: [w530 w539] -> w521
          tunnel: w512 -> [_ w535]
          tunnel: w518 -> [_ w534]
          tunnel: w513 -> [w530 w536]
          tunnel: w514 -> [_ w532]
          frame False {
          }
          frame True {
            n191 = invoke class="Tree (strict)" method="Edit Tree Items.Move Item"(reference=w548, error in=w536, "tag"=w546, "New Parent"=w544, "New Position"=w532) -> (error out=w537:errorcluster)  [unwired: 2 in, 6 out]
            n192 = Bundle By Name(cluster=T15 {"node ref"=refnum, "new parent"=refnum, "Position"=0} ("Cluster"), "new parent"=w534, "node ref"=w535, "Position"=w532) -> (w542:T15)
            n193 = Flatten To String(anything=w542, error in (no error)=w537) -> (data string=w541:string, error out=w538:errorcluster)  [unwired: 2 in, 1 out]
            n194 = call <vilib>:"Send Local Message.vi"("message queue in"=w543, "message name"="Move", "message value"=w541, "error in"=w538) -> ("message queue out"=w540:T11, "error out"=w539:errorcluster)  [unwired: 9 in, 1 out]
          }
        }
        n195 = event-data("Accepted?"=w528) -> ()  [unwired: 1 in, 1 out]
      }
      event "Exit": Value Change {
        # "Exit the application                                           >> Stop this message generator loop    Cleaning errors if the other loop stop this one"
        n196 = event-data() -> ()  [unwired: 1 in, 1 out]
        n197 = call <vilib>:"Send Local Message.vi"("message queue in"=w553, "message name"="Close", "error in"=w551) -> ("message queue out"=w549:T11, "error out"=w554:errorcluster)  [unwired: 10 in, 1 out]
        n198 = call <vilib>:"Clear Errors.vi"("error in (no error)"=w554) -> ("error out"=w550:errorcluster)  [unwired: 5 in, 1 out]
      }
      event "View": Drag Starting? {
        n199 = event-data() -> ("Data"=w566:T20, "CtlRef"=w568:refnum<vi>, "Coords"=w567:T19)  [unwired: 1 in]
        n200 = invoke class="Tree (strict)" method="Point To Row Column"(reference=w568, error in=w559, "Point"=w567) -> (error out=w558:errorcluster, "Tag"=w565:string)  [unwired: 5 in, 6 out]
        n201 = call <vilib>:"IDtoNode.vi"("error in"=w558, "ID"=w565) -> ("error out"=w557:errorcluster, "invalid Id"=w564:bool, "node ref"=w563:T2)  [unwired: 7 in]
        n202 = case shown="False" w564 {
          tunnel: w563 -> [w576 _]
          tunnel: [w573 TRUE ("Removable")] -> w561
          tunnel: w557 -> [w572 w582]
          tunnel: [w569 w582] -> w556
          frame False {
            n203 = in-place {
              in-place-border: [w579] -> w575
              in-place-border: w572 -> [w578]
              in-place-border: [w577] -> w571
              n204 = in-place-dvr #4(w576) -> (w581:refnum<class "NISE_CEF_Node.lvclass">)  [unwired: 1 out]
              n205 = call-dynamic "EditOptions.vi"("error in"=w578, "node in"=w581) -> ("error out"=w577:errorcluster, "edit options"=w579:T21, "node out"=w580:refnum<class "NISE_CEF_Node.lvclass">)  [unwired: 6 in, 1 out]
              n206 = in-place-dvr #4(w580) -> (w570:errorcluster)  [unwired: 1 out]
            }
            n207 = Unbundle By Name(w575) -> ("movable"=w574:bool)
            n208 = Merge Errors(w570, w571) -> (w569:errorcluster)
            n209 = Not(x=w574) -> (.not. x?=w573:bool)
          }
          frame True {
          }
        }
        n210 = event-data("Data"=w566, "Drag Mode"=enum32{"copy or move", "copy only", "move only"}."move only", "Discard?"=w561) -> ()  [unwired: 1 in, 1 out]
      }
      event "View": Value Change {
        n211 = event-data() -> ("NewVal"=w587:string)  [unwired: 1 in]
        n212 = call <vilib>:"Send Local Message.vi"("message queue in"=w589, "message name"="ActivateNode" ("Message Name"), "message value"=w587, "error in"=w584) -> ("message queue out"=w586:T11, "error out"=w585:errorcluster)  [unwired: 9 in, 1 out]
      }
      event "View": event type 3.0.xa000003a {
        n213 = event-data() -> ("CtlRef"=w599:refnum<vi>, "Coords"=w597:T19)  [unwired: 1 in]
        n214 = invoke class="Tree (strict)" method="Point To Row Column"(reference=w599, error in=w595, "Point"=w597) -> (reference out=w598:refnum<vi>, error out=w594:errorcluster, "Tag"=w592:string)  [unwired: 5 in, 5 out]
        n215 = call <vilib>:"ValidDragDrop.vi"("error in"=w594, "Reorder"=TRUE, "drag over"=w592, "Tree Ref in"=w598) -> ("Error Out"=w593:errorcluster, "Accepted"=w591:bool)  [unwired: 6 out]
        n216 = event-data("Accepted?"=w591) -> ()  [unwired: 1 in, 1 out]
      }
      event Panel Close? {
        # "Intercepts the upper right close panel operation to allow a smooth shutdown as opposed to immediately killing the app."
        n217 = event-data() -> ()  [unwired: 1 in, 1 out]
        n218 = call <vilib>:"Send Local Message.vi"("message queue in"=w604, "message name"="Close?", "error in"=w601) -> ("message queue out"=w602:T11, "error out"=w600:errorcluster)  [unwired: 10 in, 1 out]
        n219 = event-data("Discard?"=TRUE) -> ()  [unwired: 1 in, 1 out]
      }
      event Menu Selection (User) {
        n220 = event-data() -> ("ItemTag"=w606:string, "ItemPath"=w611:string)  [unwired: 1 in]
        n221 = case shown="\"_File:_Exit\"" w611 {
          selector: w611 -> [w615 _ _ _ _ _ _]
          tunnel: w610 -> [w620 w625 w630 w635 w640 w645 w650]
          tunnel: [w620 w621 w626 w631 w636 w641 w646] -> w609
          tunnel: w608 -> [w617 w623 w628 w633 w638 w643 w648]
          tunnel: [w616 w622 w627 w632 w637 w642 w647] -> w607
          tunnel: w606 -> [w614 _ _ _ _ _ _]
          frame Default {
            n222 = Concatenate Strings(w614, "::" ("string"), w615) -> (w613:string)
            n223 = call <vilib>:"error generator.vi"("error in"=w617, "source"="configuration tool main.vi", "append error message"=w613, "error code (0)"=538506) -> ("error out"=w616:errorcluster)  [unwired: 5 in]
          }
          frame "_File:_New" {
            n224 = call <vilib>:"Send Local Message.vi"("message queue in"=w625, "message name"="New?" ("Message Name"), "error in"=w623) -> ("message queue out"=w621:T11, "error out"=w622:errorcluster)  [unwired: 10 in, 1 out]
          }
          frame "_File:_Open" {
            n225 = call <vilib>:"Send Local Message.vi"("message queue in"=w630, "message name"="Open?" ("Message Name"), "error in"=w628) -> ("message queue out"=w626:T11, "error out"=w627:errorcluster)  [unwired: 10 in, 1 out]
          }
          frame "_File:_Save" {
            n226 = call <vilib>:"Send Local Message.vi"("message queue in"=w635, "message name"="Save" ("Message Name"), "error in"=w633) -> ("message queue out"=w631:T11, "error out"=w632:errorcluster)  [unwired: 10 in, 1 out]
          }
          frame "_File:Save As..." {
            n227 = call <vilib>:"Send Local Message.vi"("message queue in"=w640, "message name"="SaveAs" ("Message Name"), "error in"=w638) -> ("message queue out"=w636:T11, "error out"=w637:errorcluster)  [unwired: 10 in, 1 out]
          }
          frame "_File:_Build" {
            n228 = call <vilib>:"Send Local Message.vi"("message queue in"=w645, "message name"="Build" ("Message Name"), "error in"=w643) -> ("message queue out"=w641:T11, "error out"=w642:errorcluster)  [unwired: 10 in, 1 out]
          }
          frame "_File:_Exit" {
            n229 = call <vilib>:"Send Local Message.vi"("message queue in"=w650, "message name"="Close?" ("Message Name"), "error in"=w648) -> ("message queue out"=w646:T11, "error out"=w647:errorcluster)  [unwired: 10 in, 1 out]
          }
        }
      }
      event User Event {
        n230 = event-data() -> ("node ref"=w651:T2)  [unwired: 1 in]
        n231 = call <vilib>:"NodetoID.vi"("node ref"=w651) -> ("ID"=w654:string)  [unwired: 9 in, 1 out]
        n232 = call <vilib>:"Send Local Message.vi"("message queue in"=w652, "message name"="NodeDataChange", "message value"=w654) -> ("message queue out"=w653:T11)  [unwired: 10 in, 2 out]
      }
    }
    n233 = call "Error.vi"("error in (no error)"=w435, "message queue in"=w436) -> ()  [unwired: 9 in, 1 out]
  }
  n234 = Unregister For Events(event registration refnum=w8) -> (error out=w9:errorcluster)  [unwired: 1 in]
  n235 = Merge Errors(w9, w14) -> (w10:errorcluster)
  n236 = call <vilib>:"DestroyStandardEvents.vi"("error in"=w10, "standard events"=w13) -> ()  [unwired: 9 in, 1 out]
